vi "FA_GetShared Variables.vi"(8 "Error In":errorcluster) -> (0 "Error Out":errorcluster, 3 "Shared Variable":T1)   [LabVIEW 2014]
doc: "Retrieves the shared variable XML information from file and returns the shared variable typdef"
uses:
  FA_SharedVariables.ctl
  FA_LocalStore API/source/VI Source/FA_LSSpecialTypes.ctl
  FA_LocalStore API/source/VI Source/FA_LocalStore.lvlib
  FA_NativeTypes API/source/VI Source/FA_NativeTypes.lvlib
  FA_SharedVariables.lvlib
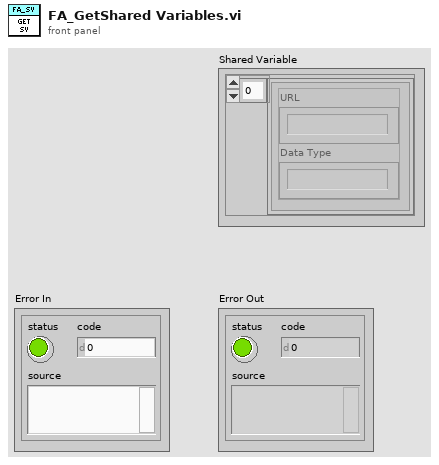
[diagram p1: front panel]
types:
  T1 = typedef "FA_SharedVariables.lvlib/FA_SharedVariables.ctl" = cluster{"Shared Variables":cluster{"URL":string, "Data Type":string}[]}
  T2 = typedef "FA_LocalStore.lvlib/FA_LSSpecialTypes.ctl" = string
  T3 = typedef "FA_NativeTypes.lvlib/FA_Config.ctl" = cluster{"Id":string, "Name":T2, "Parameter":cluster{"Name":string, "Value":string}[], "Account":string, "CreateDate":string, "LastModified":string}
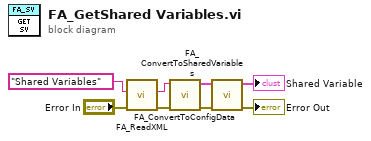
[diagram p0: block diagram]
diagram:
  n1 = call "FA_ReadXML.vi"("Error In"="Error In", "Special Type"=T2 "Shared Variables") -> ("Error Out"=w6:errorcluster, "XML String"=w5:string)  [unwired: 6 in]
  n2 = call "FA_ConvertToConfigData.vi"("Error In"=w6, "XML String"=w5) -> ("Error Out"=w4:errorcluster, "ConfigData"=w3:T3)  [unwired: 8 in]
  n3 = call "FA_ConvertToSharedVariables.vi"("Error In"=w4, "Config"=w3) -> ("Error Out"=→"Error Out":errorcluster, "SV"=→"Shared Variable":T1)  [unwired: 8 in]
